vi "StopOnSight.vi"() -> ()   [LabVIEW 2013]
uses:
  <vilib>/Platform/TimedLoop/XDataNode/timing_clust.ctl
  <vilib>/Platform/TimedLoop/XDataNode/nitl_modes.ctl
  <vilib>/Platform/TimedLoop/XDataNode/wakeup.ctl
  <vilib>/Instr/_visa.llb/VISA Configure Serial Port (Instr).vi
  <vilib>/FPGAPlugInAG/sbRIO-9642/niLvFpga_Open_sbRIO-9642.vi
  <vilib>/rvi/interface/common/dynamic/niFpgaDynamicAddResources.vi
  <vilib>/rvi/interface/common/niFpgaWaitOnOcc.vi
  <vilib>/Utility/error.llb/Error Cluster From Error Code.vi
  <vilib>/rvi/errors/niLvFpgaAdjustHostInterfaceError.vi
  <vilib>/Platform/TimedLoop/XDataNode/XDataNode.xnode
  <vilib>/rvi/interface/nirviOpenFPGA/nirviOpenFPGA.xnode
  FPGA Bitfiles/NatesProject1_FPGATarget_FPGAConfig_gDHlPw7zMRU.lvbitx
  FPGA Config.vi
  <vilib>/rvi/interface/nirviReadWriteControl/nirviReadWriteControl.xnode
  <vilib>/Platform/TimedLoop/XDataNode/XDNodeRunTimeDep.lvlib
  NiFpgaLv.dll
  <vilib>/rvi/interface/Simulation/niFpgaSimulationCallBeginRW.vi
panel:
  in  "Speed(%)":i32(knob) scale=0.0..100.0
  in  "Stop Distance":dbl(slide) scale=0.1..1.5
  out "error out":errorcluster
  out "Distance\n(cm)":dbl(slide) scale=0.0..2.5
  out "ModA/AI0":fxp<+/-,26,5>
  in  "VISA resource name":refnum<visa-resource-name>
  in  "stop":bool
  out "write buffer":string
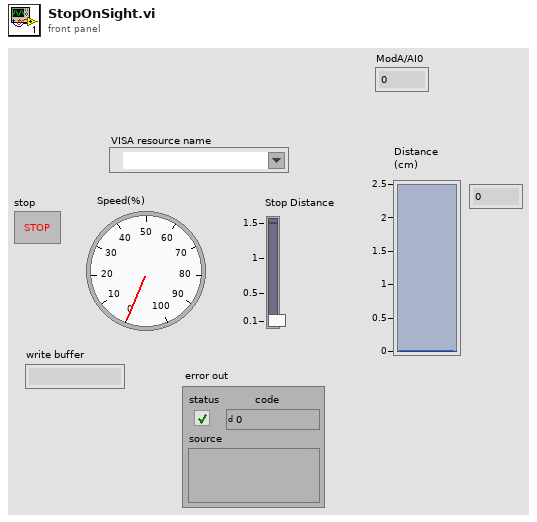
[diagram p1: front panel]
types:
  T1 = typedef "XDNodeRunTimeDep.lvlib/timing_clust.ctl" = cluster{"Expected End [f-1]":u64, "Actual End [f-1]":u64, "Finished Late? [f-1]":bool, "Expected End [i-1]":u64, "Actual End [i-1]":u64, "Finished Late? [i-1]":bool, "Expected Start [i]":u64, "Actual Start [i]":u64, "Expected Start [f]":u64, "Actual Start [f]":u64, "Source Name":string, "Structure Name":string, "Period":i64, "Deadline":i64, "Offset":i64, "Start":i64, "Priority":i32, "Timeout":i32, "Mode":T2, "Wakeup Reason":T3, "Error":errorcluster, "Source Type":string, "Secondary Source Type":string, "Global End Time":u64, "Global Start Time":u64, "Frame Duration":u64, "Iteration Duration":u64, "Assigned CPU":i32, "I/O Scan Engine Mode":u32}
  T2 = typedef "XDNodeRunTimeDep.lvlib/nitl_modes.ctl" = enum32{"No Change", "Process missed periods, maintain original phase", "Discard missed periods, maintain original phase", "Process missed periods, ignore original phase", "Discard missed periods, ignore original phase"}
  T3 = typedef "XDNodeRunTimeDep.lvlib/wakeup.ctl" = enum32{"Normal", "Aborted", "Asynchronous wakeup", "Timing source error", "Timed loop error", "Timeout"}
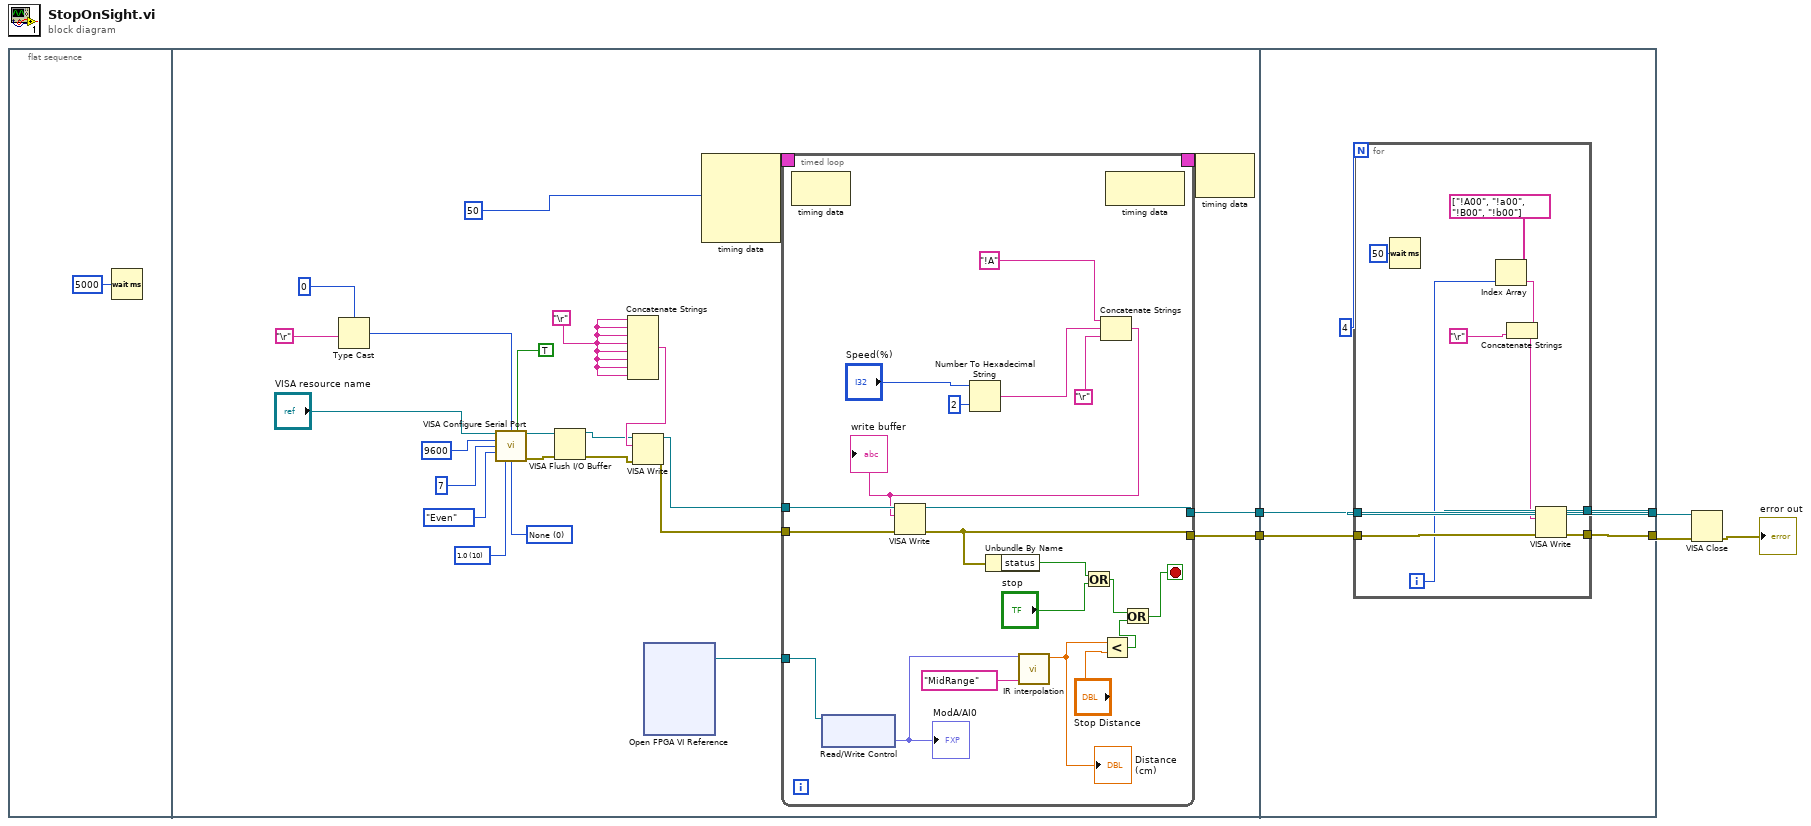
[diagram p0: block diagram]
diagram:
  n1 = flat-sequence {
    tunnel: [w9] -> w5
    tunnel: [w8] -> w4
    tunnel: [w58] -> w2
    tunnel: [w59] -> w3
    tunnel: w5 -> [w61]
    tunnel: w4 -> [w60]
    frame #0 {
      n2 = Wait (ms)(milliseconds to wait=u32 5000) -> ()  [unwired: 1 out]
    }
    frame #1 {
      w15 = "\r"
      w22 = u16 0 items=["None", "XON/XOFF", "RTS/CTS", "XON/XOFF & RTS/CTS", "DTR/DSR", "XON/XOFF & DTR/DSR"] ("flow control (0:none)")
      w23 = u16 10 items=["1.0"=10, "1.5"=15, "2.0"=20] ("stop bits (10: 1 bit)")
      n3 = Type Cast(type=0, x="\r") -> (*(type *) &x=w18:i32)
      n4 = call-poly "VISA Configure Serial Port"("VISA resource name"="VISA resource name", "termination char\n(0xA = '\\n' = LF)"=w18, "Enable Termination\nChar (T)"=TRUE ("Enable Termination\nChar (T)"), "baud rate (9600)"=u32 9600, "data bits (8)"=u16 7, "parity (0:none)"=enum16{"None", "Odd", "Even", "Mark", "Space"}."Even", "stop bits (10: 1 bit)"=w23, "flow control (0:none)"=w22) -> ("VISA resource name out"=w16:refnum<visa-resource-name>, "error out"=w17:errorcluster)  [unwired: 6 in]
      n5 = VISA Flush I/O Buffer(VISA resource name=w16, error in (no error)=w17) -> (VISA resource name out=w13:refnum<visa-resource-name>, error out=w12:errorcluster)  [unwired: 1 in]
      n6 = Concatenate Strings(w15, w15, w15, w15, w15, w15, w15, w15) -> (w14:string)
      n7 = VISA Write(VISA resource name=w13, write buffer=w14, error in (no error)=w12) -> (VISA resource name out=w11:refnum<visa-resource-name>, error out=w10:errorcluster)  [unwired: 1 out]
      n8 = xnode "Open FPGA VI Reference"() -> ("FPGA VI Reference Out"=w7:refnum<k20>)  [unwired: 2 in, 1 out]
      n9 = node-c288(i64 50 ("Period")) -> (w30:T1)  [unwired: 3 in]
      n10 = timed-loop {
        timing: w30 -> [_]
        timing-out: [_] -> w29
        tunnel: w11 -> [w47]
        tunnel: w10 -> [w46]
        tunnel: [w41] -> w9
        tunnel: [w42] -> w8
        tunnel: w7 -> [w37]
        stop <- w38 stop-if-true
        n11 = node-c288() -> ()  [unwired: 1 in, 1 out]
        n12 = xnode "Read/Write Control"("FPGA VI Reference In"=w37) -> ("ModA/AI1"=w33:fxp<+/-,26,5>)  [unwired: 1 in, 2 out]
        "ModA/AI0" <- w33
        n13 = Number To Hexadecimal String(1:i16 2 ("width (-)"), 2:"Speed(%)") -> (0:w49:string)
        n14 = call "IR interpolation.vi"("IR Sensor Type"="MidRange", "x value"=w33) -> ("interpolation value"=w31:dbl)  [unwired: 9 in]
        "Distance\n(cm)" <- w31
        n15 = Concatenate Strings("!A", w49, "\r") -> (w45:string)
        "write buffer" <- w45
        n16 = VISA Write(VISA resource name=w47, write buffer=w45, error in (no error)=w46) -> (VISA resource name out=w41:refnum<visa-resource-name>, error out=w42:errorcluster)  [unwired: 1 out]
        n17 = Unbundle By Name(w42) -> ("status"=w44:bool)
        n18 = Or(x=w44, y="stop") -> (x .or. y?=w39:bool)
        n19 = Less?(x=w31, y="Stop Distance") -> (x < y?=w36:bool)
        n20 = node-c288() -> ()  [unwired: 1 in, 1 out]
        n21 = Or(x=w39, y=w36) -> (x .or. y?=w38:bool)
      }
      n22 = node-c288(w29) -> ()  [unwired: 1 out]
    }
    frame #2 {
      n23 = for {
        N: 4 -> [_]
        tunnel: w61 -> [w71]
        tunnel: w60 -> [w70]
        tunnel: [w69] -> w59
        tunnel: [w68] -> w58
        i -> [w66]
        n24 = Wait (ms)(milliseconds to wait=u32 50) -> ()  [unwired: 1 out]
        n25 = Index Array(array=string[] ["!A00", "!a00", "!B00", "!b00"], index=w66) -> (element=w64:string)
        n26 = Concatenate Strings(w64, "\r") -> (w62:string)
        n27 = VISA Write(VISA resource name=w71, write buffer=w62, error in (no error)=w70) -> (VISA resource name out=w69:refnum<visa-resource-name>, error out=w68:errorcluster)  [unwired: 1 out]
      }
    }
  }
  n28 = VISA Close(VISA resource name=w3, error in (no error)=w2) -> (error out=→"error out":errorcluster)
